vi "RunOven.vi"   [LabVIEW 2012]
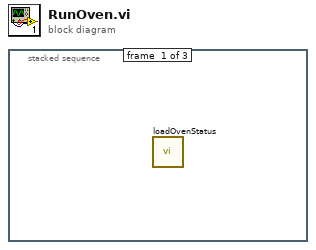
[diagram p0: block diagram]
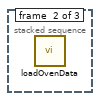
[diagram p2: hidden frame]
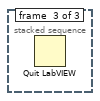
[diagram p3: hidden frame]
diagram:
  n1 = stacked-sequence {
    frame #0 {
      n2 = call "loadOvenStatus.vi"() -> ()  [unwired: 12 in]
    }
    frame #1 {
      n3 = call "loadOvenData.vi"() -> ()  [unwired: 12 in]
    }
    frame #2 {
      n4 = Quit LabVIEW() -> ()  [unwired: 1 in]
    }
  }
